vi "Write Problem.vi"(6 "Overwrite without confirmation? (F)":bool, 7 "floating point precision (6)":i16=6, 8 "error in (no error)":errorcluster, 10 "svm_problem":T1, 11 "file path (use dialog)":path=path "") -> (0 "error out":errorcluster)   [LabVIEW 2015]
uses:
  LibSVM Sparse/Wrapper API/Controls/svm_problem.ctl
  LibSVM Sparse/Wrapper API/Controls/svm_node.ctl
  <userlib>/_OpenG.lib/file/file.llb/Valid Path - Traditional__ogtk.vi
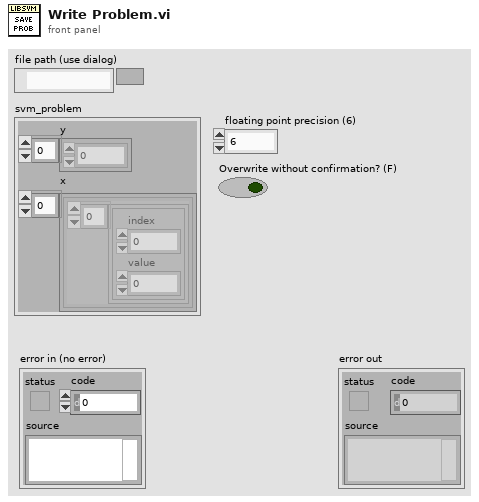
[diagram p1: front panel]
types:
  T1 = typedef "svm_problem.ctl" = cluster{"y":dbl[], "x":cluster{T2[]}[]}
  T2 = typedef "svm_node.ctl" = cluster{"index":i32, "value":dbl}
  T3 = enum16{"open", "replace", "create", "open or create", "replace or create", "replace or create with confirmation"}
  T4 = enum16{"Native", "Native Command Line", "UNIX", "Macintosh", "DOS"}
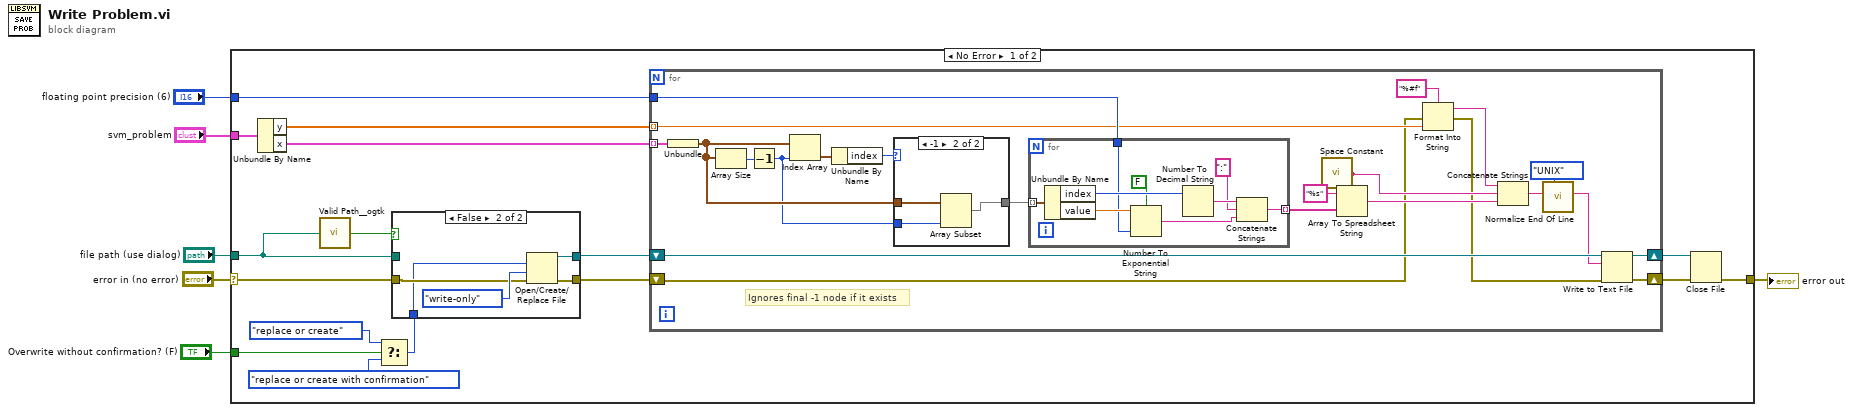
[diagram p0: block diagram]
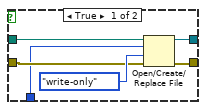
[diagram p3: hidden frame]
diagram:
  n1 = case shown="No Error" "error in (no error)" {
    selector: "error in (no error)" -> [w22 w70]
    tunnel: [w7 w70] -> w6
    tunnel: "svm_problem" -> [w15 _]
    tunnel: "file path (use dialog)" -> [w16 _]
    tunnel: "Overwrite without confirmation? (F)" -> [w20 _]
    tunnel: "floating point precision (6)" -> [w10 _]
    frame No Error {
      n2 = Unbundle By Name(w15) -> ("y"=w13:dbl[], "x"=w14:cluster{T2[]}[])
      n3 = call-poly <userlib>:"Valid Path__ogtk.vi"("path"=w16) -> ("valid"=w17:bool)
      n4 = Select(t=T3."replace or create" ("operation (0:open)"), s=w20, f=T3."replace or create with confirmation" ("operation (0:open)")) -> (s? t:f=w18:T3)
      n5 = case shown="False" w17 {
        tunnel: w22 -> [w63 w68]
        tunnel: [w62 w67] -> w12
        tunnel: [w61 w66] -> w11
        tunnel: w18 -> [w60 w65]
        tunnel: w16 -> [w59 _]
        frame True {
          n6 = Open/Create/Replace File(file path (use dialog)=w59, error in=w63, operation (0:open)=w60, access (0:read/write)=enum16{"read/write", "read-only", "write-only"}."write-only") -> (refnum out=w61:refnum<file>, error out=w62:errorcluster)  [unwired: 2 in, 1 out]
        }
        frame False {
          n7 = Open/Create/Replace File(error in=w68, operation (0:open)=w65, access (0:read/write)=enum16{"read/write", "read-only", "write-only"}."write-only") -> (refnum out=w66:refnum<file>, error out=w67:errorcluster)  [unwired: 3 in, 1 out]
        }
      }
      n8 = for {
        tunnel: w14 -> [w45] mode=indexing
        tunnel: w13 -> [w27] mode=indexing
        tunnel: w10 -> [w43]
        shift-right: [w39] -> w9
        shift-left: w11 -> [w44]
        shift-right: [w38] -> w8
        shift-left: w12 -> [w26]
        # "Ignores final -1 node if it exists"
        n9 = Unbundle(w45) -> (w29:T2[])
        n10 = Array Size(array=w29) -> (size(s)=w33:i32)
        n11 = Decrement(x=w33) -> (x-1=w28:i32)
        n12 = Index Array(array=w29, index=w28) -> (element=w32:T2)
        n13 = Unbundle By Name(w32) -> ("index"=w31:i32)
        n14 = case shown="-1" w31 {
          tunnel: [w46 w48] -> w30
          tunnel: w29 -> [w46 w49]
          tunnel: w28 -> [_ w47]
          frame Default {
          }
          frame -1 {
            n15 = Array Subset(array=w49, length=w47) -> (w48:T2[])  [unwired: 1 in]
          }
        }
        n16 = for {
          tunnel: w30 -> [w58] mode=indexing
          tunnel: w43 -> [w51]
          tunnel: [w54] -> w42 mode=indexing
          n17 = Unbundle By Name(w58) -> ("index"=w57:i32, "value"=w53:dbl)
          n18 = Number To Exponential String(number=w53, precision (6)=w51, 1:FALSE ("use system decimal point (T)")) -> (E-format string=w52:string)  [unwired: 1 in]
          n19 = Number To Decimal String(number=w57) -> (decimal integer string=w56:string)  [unwired: 1 in]
          n20 = Concatenate Strings(w56, ":" ("string"), w52) -> (w54:string)
        }
        n21 = call <vilib>:"Space Constant.vi"() -> ("String"=w40:string)
        n22 = Array To Spreadsheet String(delimiter (Tab)=w40, array=w42, 3:"%s" ("format string")) -> (spreadsheet string=w36:string)
        n23 = Format Into String(format string="%#f", error in=w26, w27) -> (resulting string=w24:string, error out=w25:errorcluster)  [unwired: 1 in]
        n24 = Concatenate Strings(w24, w40, w36) -> (w35:string)
        n25 = call <vilib>:"Normalize End Of Line.vi"("end of line (Native)"=T4."UNIX", "string in"=w35) -> ("string out"=w34:string)  [unwired: 6 in]
        n26 = Write to Text File(file (use dialog)=w44, text=w34, error in=w25) -> (refnum out=w39:refnum<file>, error out=w38:errorcluster)  [unwired: 1 in, 1 out]
      }
      n27 = Close File(refnum=w9, error in=w8) -> (error out=w7:errorcluster)  [unwired: 1 out]
    }
    frame Error {
    }
  }
  "error out" <- w6
